vi "subVi_extr_serv.vi"(1 "Servicios_Edif":bool[](array[boolean])) -> (0 "serv":string)   [LabVIEW 2017]
panel:
  # "a  Luz"
  # "b  Aire"
  # "c  Proyector"
  # "d  Agua"
  # "e  Acceso"
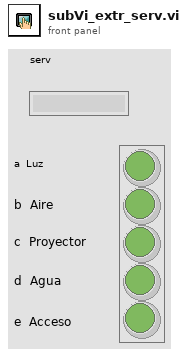
[diagram p1: front panel]
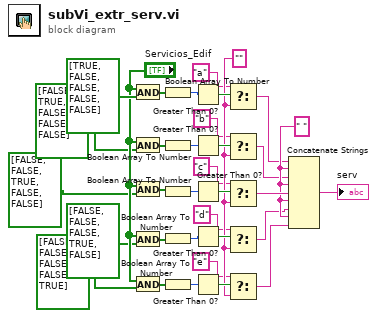
[diagram p0: block diagram]
diagram:
  w12 = ""
  w5 = " "
  n1 = And(x="Servicios_Edif", y=bool[] [TRUE, FALSE, FALSE, FALSE, FALSE]) -> (x .and. y?=w32:bool[])
  n2 = And(x="Servicios_Edif", y=bool[] [FALSE, TRUE, FALSE, FALSE, FALSE]) -> (x .and. y?=w31:bool[])
  n3 = And(x="Servicios_Edif", y=bool[] [FALSE, FALSE, TRUE, FALSE, FALSE]) -> (x .and. y?=w30:bool[])
  n4 = And(x="Servicios_Edif", y=bool[] [FALSE, FALSE, FALSE, TRUE, FALSE]) -> (x .and. y?=w29:bool[])
  n5 = And(x="Servicios_Edif", y=bool[] [FALSE, FALSE, FALSE, FALSE, TRUE]) -> (x .and. y?=w28:bool[])
  n6 = Boolean Array To Number(Boolean array=w32) -> (number=w27:u32)
  n7 = Boolean Array To Number(Boolean array=w31) -> (number=w26:u32)
  n8 = Boolean Array To Number(Boolean array=w30) -> (number=w25:u32)
  n9 = Boolean Array To Number(Boolean array=w29) -> (number=w24:u32)
  n10 = Boolean Array To Number(Boolean array=w28) -> (number=w23:u32)
  n11 = Greater Than 0?(x=w27) -> (x > 0?=w17:bool)
  n12 = Greater Than 0?(x=w26) -> (x > 0?=w16:bool)
  n13 = Greater Than 0?(x=w25) -> (x > 0?=w15:bool)
  n14 = Greater Than 0?(x=w24) -> (x > 0?=w14:bool)
  n15 = Greater Than 0?(x=w23) -> (x > 0?=w13:bool)
  n16 = Select(t="a", s=w17, f=w12) -> (s? t:f=w4:string)
  n17 = Select(t="b", s=w16, f=w12) -> (s? t:f=w3:string)
  n18 = Select(t="c", s=w15, f=w12) -> (s? t:f=w6:string)
  n19 = Select(t="d", s=w14, f=w12) -> (s? t:f=w2:string)
  n20 = Select(t="e", s=w13, f=w12) -> (s? t:f=w1:string)
  n21 = Concatenate Strings(w4, w5, w3, w5, w6, w5, w2, w5, w1) -> (→"serv":string)
